vi "Write Ball.vi"(8 "error in (no error)":errorcluster, 10 "RT_Game.lvlib:PongBall.lvclass":refnum<class "PongBall.lvclass">, 11 "Bouncer in":refnum<class "Bouncer.lvclass">) -> (0 "error out":errorcluster, 3 "Bouncer out":refnum<class "Bouncer.lvclass">)   [LabVIEW 2019, in "RT_Game.lvlib" / "Bouncer.lvclass"]
uses:
  Bouncer.lvclass
  PongBall/PongBall.lvclass
  Bouncer.lvclass/Bouncer.ctl
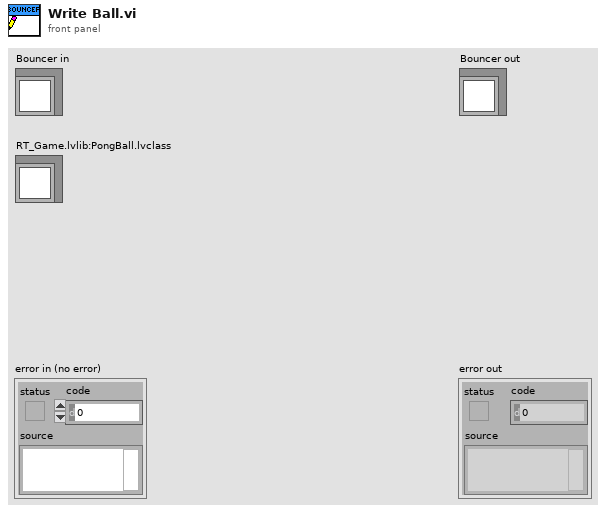
[diagram p1: front panel]
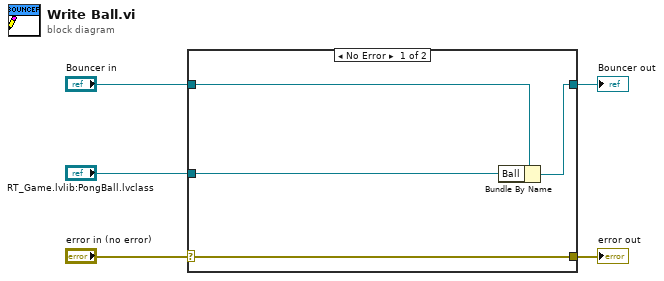
[diagram p0: block diagram]
diagram:
  n1 = case shown="No Error" "error in (no error)" {
    selector: "error in (no error)" -> [w9 w10]
    tunnel: [w9 w10] -> w4
    tunnel: [w7 w11] -> w2
    tunnel: "Bouncer in" -> [w8 w11]
    tunnel: "RT_Game.lvlib:PongBall.lvclass" -> [w6 _]
    frame No Error {
      n2 = Bundle By Name(cluster=w8, "Ball"=w6) -> (w7:refnum<class "Bouncer.lvclass">)
    }
    frame Error {
    }
  }
  "error out" <- w4
  "Bouncer out" <- w2
